vi "Check config IPS.vi"(3 "error in (no error)":errorcluster, 4 "input cluster":T1 {"MaxLambdaCurrent [A]" format="%.2f"; "LambdaRates [A/min]" format="%.2f"; "MaxNormalCurrent [A]" format="%.2f"; "StabilitySetting [%]" format="%.2f"; "FieldCurrentRatio [T/A]" format="%.2f"; "SwitchWaitTime [s]" format="%.2f"; "SwitchHtrCurrent [mA]" format="%.2f"; "TrainRates [A/min]" format="%.2f"; "NormalRates [A/min]" format="%.2f"; "Breakpts [A]" format="%.2f"}, 5 "VISA session":refnum<visa-resource-name>="GPIB0::22::INSTR") -> (0 "error out":errorcluster, 1 "output cluster":T1 {"MaxLambdaCurrent [A]" format="%.2f"; "LambdaRates [A/min]" format="%.2f"; "MaxNormalCurrent [A]" format="%.2f"; "StabilitySetting [%]" format="%.2f"; "FieldCurrentRatio [T/A]" format="%.2f"; "SwitchWaitTime [s]" format="%.2f"; "SwitchHtrCurrent [mA]" format="%.2f"; "TrainRates [A/min]" format="%.2f"; "NormalRates [A/min]" format="%.2f"; "Breakpts [A]" format="%.2f"}, 2 "VISA session 2":refnum<visa-resource-name>)   [LabVIEW 2020]
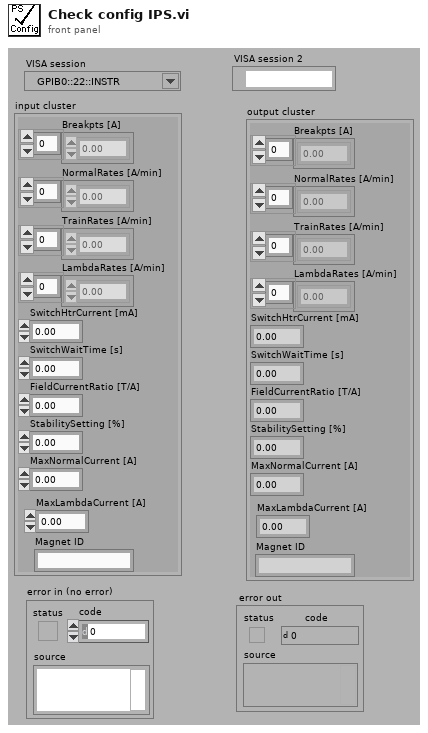
[diagram p1: front panel]
types:
  T1 = cluster{"Breakpts [A]":dbl[], "NormalRates [A/min]":dbl[], "TrainRates [A/min]":dbl[], "SwitchHtrCurrent [mA]":dbl, "SwitchWaitTime [s]":dbl, "FieldCurrentRatio [T/A]":dbl, "StabilitySetting [%]":dbl, "MaxNormalCurrent [A]":dbl, "Magnet ID":string, "LambdaRates [A/min]":dbl[], "MaxLambdaCurrent [A]":dbl}
  T2 = enum16{"SwitchHtrCurrent", "SwitchWaitTime", "FieldCurrentRatio", "StabilitySetting", "MaxNormalCurrent", "MaxLambdaCurrent"}
  T3 = enum16{"Normal", "Train", "Lambda", "Train & Lambda"}
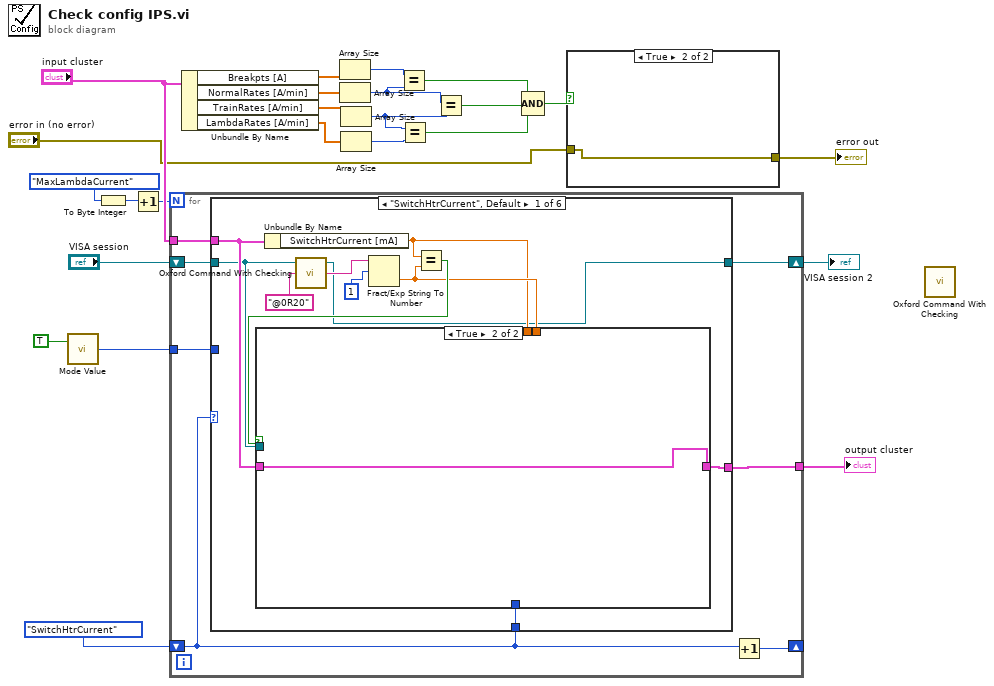
[diagram p0: block diagram]
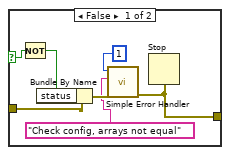
[diagram p2: hidden frame]
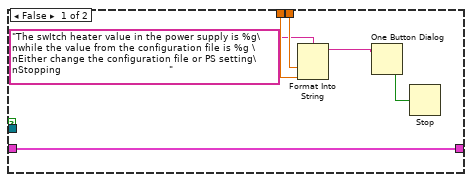
[diagram p3: hidden frame]
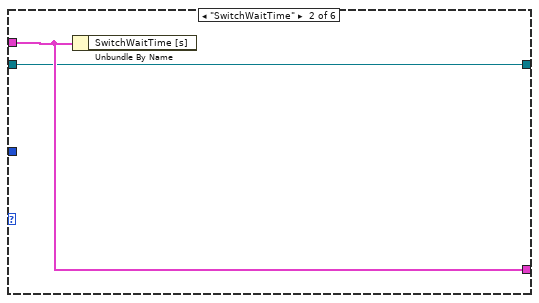
[diagram p4: hidden frame]
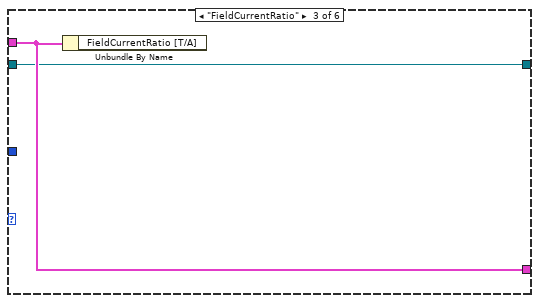
[diagram p5: hidden frame]
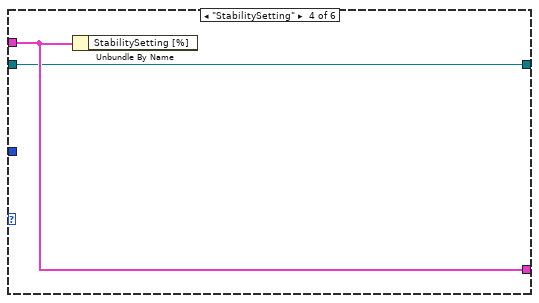
[diagram p6: hidden frame]
diagram:
  # "x"
  n1 = call "Mode Value.vi"("Read/Write this vi"=TRUE) -> ("Mode Out"=w7:T3)  [unwired: 1 in]
  n2 = To Byte Integer(number=T2."MaxLambdaCurrent") -> (8bit integer=w4:i8)
  n3 = Increment(x=w4) -> (x+1=w3:i8)
  n4 = for {
    N: w3 -> [_]
    tunnel: "input cluster" -> [w30]
    tunnel: [w29] -> w6
    shift-right: [w28] -> _
    shift-left: T2."SwitchHtrCurrent" -> [w27]
    tunnel: w7 -> [w26]
    shift-right: [w25] -> w1
    shift-left: "VISA session" -> [w31]
    n5 = case shown="\"SwitchHtrCurrent\", Default" w27 {
      tunnel: w31 -> [w36 w50 w52 w54 w56 w58]
      tunnel: w30 -> [w39 w51 w53 w55 w57 w59]
      tunnel: [w38 w51 w53 w55 w57 w59] -> w29
      tunnel: w27 -> [w37 _ _ _ _ _]
      tunnel: w26 -> [_ _ _ _ _ _]
      tunnel: [w32 w50 w52 w54 w56 w58] -> w25
      frame "SwitchHtrCurrent", Default {
        n6 = Unbundle By Name(w39) -> ("SwitchHtrCurrent [mA]"=w40:dbl)
        n7 = call "Oxford Command With Checking.vi"("Command"="@0R20" ("Command String"), "VISA session"=w36) -> ("String Read"=w34:string, "dup VISA session"=w32:refnum<visa-resource-name>)  [unwired: 1 in, 1 out]
        n8 = Fract/Exp String To Number(string=w34, offset=1 ("index")) -> (number=w41:dbl)  [unwired: 2 in, 1 out]
        n9 = Equal?(x=w40, y=w41) -> (x = y?=w42:bool)
        n10 = case shown="True" w42 {
          tunnel: w41 -> [w47 _]
          tunnel: w40 -> [w48 _]
          tunnel: w36 -> [_ _]
          tunnel: w39 -> [w43 w49]
          tunnel: [w43 w49] -> w38
          tunnel: w37 -> [_ _]
          frame False {
            n11 = Format Into String(format string="The swItch heater value in the power supply is %g\nwhile the value from the configuration file is %g \nEither change the configuration file or PS setting\nStopping                                    " ("message"), w47, w48) -> (resulting string=w45:string)  [unwired: 2 in, 1 out]
            n12 = One Button Dialog(message=w45) -> (true=w44:bool)  [unwired: 1 in]
            n13 = Stop(stop? (T)=w44) -> ()
          }
          frame True {
          }
        }
      }
      frame "SwitchWaitTime" {
        n14 = Unbundle By Name(w51) -> ()  [unwired: 1 out]
      }
      frame "FieldCurrentRatio" {
        n15 = Unbundle By Name(w53) -> ()  [unwired: 1 out]
      }
      frame "StabilitySetting" {
        n16 = Unbundle By Name(w55) -> ()  [unwired: 1 out]
      }
      frame "MaxNormalCurrent" {
      }
      frame "MaxLambdaCurrent" {
      }
    }
    n17 = Increment(x=w27) -> (x+1=w28:T2)
  }
  "output cluster" <- w6
  "VISA session 2" <- w1
  n18 = Unbundle By Name("input cluster") -> ("Breakpts [A]"=w22:dbl[], "NormalRates [A/min]"=w24:dbl[], "TrainRates [A/min]"=w23:dbl[], "LambdaRates [A/min]"=w16:dbl[])
  n19 = Array Size(array=w22) -> (size(s)=w21:i32)
  n20 = Array Size(array=w24) -> (size(s)=w13:i32)
  n21 = Array Size(array=w23) -> (size(s)=w14:i32)
  n22 = Array Size(array=w16) -> (size(s)=w15:i32)
  n23 = Equal?(x=w21, y=w13) -> (x = y?=w12:bool)
  n24 = Equal?(x=w14, y=w15) -> (x = y?=w10:bool)
  n25 = Equal?(x=w13, y=w14) -> (x = y?=w11:bool)
  n26 = Compound Arithmetic op=AND(w12, w11, w10) -> (w20:bool)
  n27 = case shown="True" w20 {
    selector: w20 -> [w65 _]
    tunnel: [w64 w67] -> w18
    tunnel: "error in (no error)" -> [w63 w67]
    frame False {
      n28 = Not(x=w65) -> (.not. x?=w61:bool)
      n29 = Bundle By Name(cluster=w63, "status"=w61) -> (w62:errorcluster)
      n30 = call <vilib>:"Simple Error Handler.vi"("error code (no error:0)"=1, "error source (\" \")"="Check config, arrays not equal" ("error source (\" \")"), "error in (no error)"=w62) -> ("error out"=w64:errorcluster)  [unwired: 2 in, 4 out]
      n31 = Stop(stop? (T)=w64) -> ()
    }
    frame True {
    }
  }
  "error out" <- w18
  n32 = call "Oxford Command With Checking.vi"() -> ()  [unwired: 3 in, 3 out]
